vi "Prepare map measurement.vi"(8 "error in (no error)":errorcluster, 9 "Map parameters":T3 {"Sampling rate" items=["117 ks/S"=9, "58.6 kS/s"=10, "29.3 kS/s"=11, "14.6 kS/s"=12, "7.32 kS/s"=13, "3.66 kS/s"=14, "1.83 kS/s"=15]}, 10 "ACQ parameters":T2 {"Enable output" items=["Disable", "Enable"]; "Amp_Mod [mV]" min=0.0 max=10000.0; "F_Mod [kHz]" min=0.1 max=500.0; "Filter order" min=1.0 max=9.0 step=1.0; "Time constant [ms]" min=0.0 max=1000.0}, 11 "Referencies in":T1) -> (0 "error out":errorcluster)   [LabVIEW 2024]
uses:
  Datatypes/Map parameters.ctl
  Subsystem modules/Lock-in module/ctl/OSC sampling rate.ctl
  Subsystem modules/Lock-in module/ctl/MFLI parameters.ctl
  Subsystem modules/Messenger service/Data types/Messenger referencies.ctl
  Subsystem modules/Lock-in module/ctl/MFLI_message for module.ctl
  Subsystem modules/Lock-in module/ctl/MFLI_command enum.ctl
  Subsystem modules/Temperature control module/ctl/MSG for VTI.ctl
  Subsystem modules/Temperature control module/ctl/TC commands.ctl
  Subsystem modules/Magnet module/ctl/MSG to magnet.ctl
  Subsystem modules/Magnet module/ctl/Magnet Orders.ctl
  Subsystem modules/Temperature control module/ctl/Set point.ctl
  Subsystem modules/Magnet module/ctl/SetField data.ctl
  Subsystem modules/Magnet module/ctl/Magnet mode public.ctl
  Subsystem modules/Lock-in module/ctl/MFLI_parameter and value.ctl
  Subsystem modules/Lock-in module/ctl/MFLI_node.ctl
  Subsystem modules/Lock-in module/Lock-in module.lvlib
  Subsystem modules/Temperature control module/Temperature controller.lvlib
  Subsystem modules/Magnet module/Magnet module.lvlib
  Subsystem modules/Messenger service/MessengerLib.lvlib
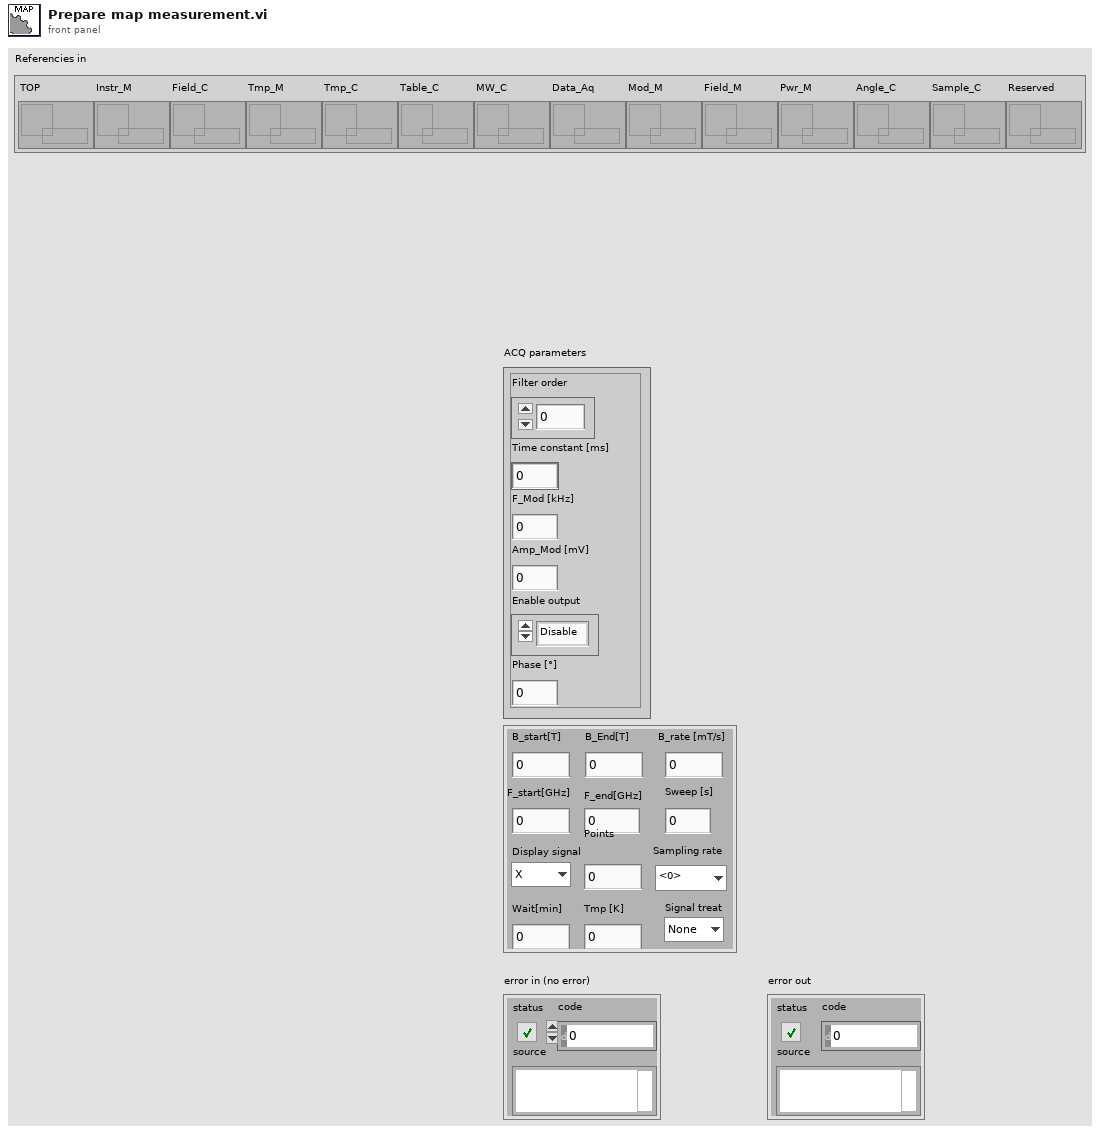
[diagram p1: front panel]
types:
  T1 = typedef "MessengerLib.lvlib/Messenger referencies.ctl" = cluster{"TOP":refnum<queue>, "Instr_M":refnum<queue>, "Field_C":refnum<queue>, "Tmp_M":refnum<queue>, "Tmp_C":refnum<queue>, "Table_C":refnum<queue>, "MW_C":refnum<queue>, "Data_Aq":refnum<queue>, "Mod_M":refnum<queue>, "Field_M":refnum<queue>, "Pwr_M":refnum<queue>, "Angle_C":refnum<queue>, "Sample_C":refnum<queue>, "Reserved":refnum<queue>}
  T2 = typedef "Lock-in module.lvlib/MFLI parameters.ctl" = cluster{"Filter order":dbl, "Time constant [ms]":dbl, "F_Mod [kHz]":dbl, "Amp_Mod [mV]":dbl, "Enable output":u16, "Phase [°]":dbl}
  T3 = typedef "Map parameters.ctl" = cluster{"B_start[T]":dbl, "B_End[T]":dbl, "B_rate [mT/s]":dbl, "F_start[GHz]":dbl, "F_end[GHz]":dbl, "Sampling rate":T4, "Tmp [K]":dbl, "Wait[min]":dbl, "Points":u32, "Display signal":enum16{"X", "Y", "R", "Phi"}, "Signal treat":enum16{"None", "Unity norm", "Mean norm", "Standardization"}, "Sweep [s]":dbl}
  T4 = typedef "OSC sampling rate.ctl" = u16
  T5 = typedef "Magnet module.lvlib/MSG to magnet.ctl" = cluster{"Order":T6, "Data":variant}
  T6 = typedef "Magnet module.lvlib/Magnet Orders.ctl" = enum16{"Ignore", "Connect", "Update", "Switch mode", "Set field", "Stop ramping", "Equalize output", "Zero output", "Flip polarity", "Blackout", "Set timer", "Eval temperatures", "Disconnect"}
  T7 = typedef "Lock-in module.lvlib/MFLI_parameter and value.ctl" = cluster{"parameter":T8, "value":dbl}
  T8 = typedef "Lock-in module.lvlib/MFLI_node.ctl" = enum16{"None", "filter_order [-]", "filter_constant [ms]", "in_diff", "in_autorange", "in_imp50", "in_AC", "osc_freq [kHz]", "out_ampl [V]", "out_autorange", "out_imp50", "enable output", "enamble ampl", "scope_enable", "scope_rate", "scope_len", "scope_trigEn", "AuxOut_amplify", "Phase_deg", "AuxOut_select"}
  T9 = typedef "Lock-in module.lvlib/MFLI_message for module.ctl" = cluster{"Command":T10, "Data":variant}
  T10 = typedef "Lock-in module.lvlib/MFLI_command enum.ctl" = enum16{"Initialize", "Update", "Set parameters", "Set module", "Set individual parameters", "Get point", "Get array", "Disconnect", "End", "Ignore"}
  T11 = typedef "Magnet module.lvlib/SetField data.ctl" = cluster{"Field [T]":dbl, "Ramp [T/s]":dbl, "Custom Ramp?":bool, "Mode":T12}
  T12 = typedef "Magnet module.lvlib/Magnet mode public.ctl" = enum16{"Persistant", "Ramping"}
  T13 = typedef "Temperature controller.lvlib/Set point.ctl" = cluster{"Heater":string, "Tmp [K]":dbl}
  T14 = typedef "Temperature controller.lvlib/MSG for VTI.ctl" = cluster{"Command":T15, "Data":variant}
  T15 = typedef "Temperature controller.lvlib/TC commands.ctl" = enum16{"Initialize", "Update", "Stop tmp change", "Set temperature", "Set point", "Disconnect", "End", "Ignore"}
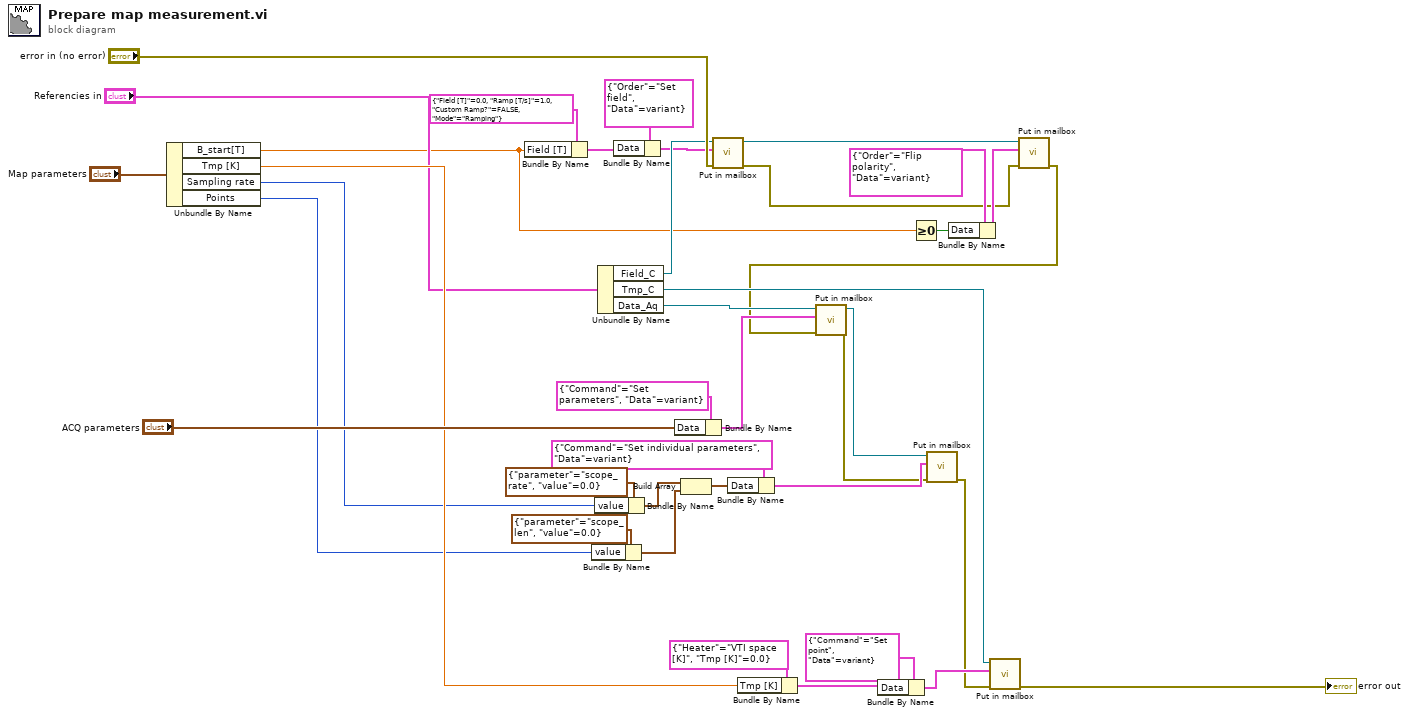
[diagram p0: block diagram]
diagram:
  n1 = Unbundle By Name("Map parameters") -> ("B_start[T]"=w3:dbl, "Tmp [K]"=w32:dbl, "Sampling rate"=w14:T4, "Points"=w13:u32)
  n2 = Bundle By Name(cluster=T11 {"Field [T]"=0.0, "Ramp [T/s]"=1.0, "Custom Ramp?"=FALSE, "Mode"=enum."Ramping"} ("Set Field"), "Field [T]"=w3) -> (w21:T11)
  n3 = Bundle By Name(cluster=T7 {"parameter"=enum."scope_len", "value"=0.0} ("element"), "value"=w13) -> (w15:T7)
  n4 = Bundle By Name(cluster=T7 {"parameter"=enum."scope_rate", "value"=0.0} ("Parameter to set"), "value"=w14) -> (w16:T7)
  n5 = Unbundle By Name("Referencies in") -> ("Field_C"=w23:refnum<queue>, "Tmp_C"=w38:refnum<queue>, "Data_Aq"=w37:refnum<queue>)
  n6 = Bundle By Name(cluster=T5 {"Order"=enum."Set field", "Data"=variant} ("MSG to magnet"), "Data"=w21) -> (w20:T5)
  n7 = Bundle By Name(cluster=T9 {"Command"=enum."Set parameters", "Data"=variant} ("MSG for  ACQ"), "Data"="ACQ parameters") -> (w22:T9)
  n8 = Build Array(w16, w15) -> (w18:T7[])
  n9 = call "Put in mailbox.vi"("error in (no error)"="error in (no error)", "Message"=w20, "Queue in"=w23) -> ("error out"=w1:errorcluster, "Queue out"=w6:refnum<queue>)  [unwired: 6 in, 1 out]
  n10 = Bundle By Name(cluster=T9 {"Command"=enum."Set individual parameters", "Data"=variant} ("MSG for  ACQ"), "Data"=w18) -> (w11:T9)
  n11 = Bundle By Name(cluster=T13 {"Heater"="VTI space [K]", "Tmp [K]"=0.0} ("Set point"), "Tmp [K]"=w32) -> (w25:T13)
  n12 = Bundle By Name(cluster=T14 {"Command"=enum."Set point", "Data"=variant} ("MSG for VTI"), "Data"=w25) -> (w24:T14)
  n13 = Greater Or Equal To 0?(x=w3) -> (x >= 0?=w4:bool)
  n14 = Bundle By Name(cluster=T5 {"Order"=enum."Flip polarity", "Data"=variant} ("MSG to magnet"), "Data"=w4) -> (w5:T5)
  n15 = call "Put in mailbox.vi"("error in (no error)"=w1, "Message"=w5, "Queue in"=w6) -> ("error out"=w2:errorcluster)  [unwired: 6 in, 2 out]
  n16 = call "Put in mailbox.vi"("error in (no error)"=w2, "Message"=w22, "Queue in"=w37) -> ("error out"=w8:errorcluster, "Queue out"=w10:refnum<queue>)  [unwired: 6 in, 1 out]
  n17 = call "Put in mailbox.vi"("error in (no error)"=w8, "Message"=w11, "Queue in"=w10) -> ("error out"=w9:errorcluster)  [unwired: 6 in, 2 out]
  n18 = call "Put in mailbox.vi"("error in (no error)"=w9, "Message"=w24, "Queue in"=w38) -> ("error out"=→"error out":errorcluster)  [unwired: 6 in, 2 out]
